vi "DrawBarPlot.vi"(0 "reference in":refnum<class "LcWebView.lvclass">, 1 "XLabels":string[](array[string]), 2 "BarPlot.Dataset":dbl[][](array[numeric]), 3 "BarPlot.DatasetLabels":string[](array[string]), 5 "Error In":errorcluster, 6 "GenericPlotOptions":T2, 7 "BarPlot.PlotColours":u32[](array[numeric]), 8 "BarPlotOptions":T1={"xLabel"="", "yLabel"="", "DisplayXLabel"=TRUE, "DisplayYLabel"=TRUE, "Stacked"=TRUE}) -> (14 "reference out":refnum<class "LcWebView.lvclass">, 19 "Error Out":errorcluster)   [LabVIEW 2020, in "LcWebView.lvclass"]
uses:
  LcWebView.lvclass
  ctrls/GenericPlotOption.ctl
  <userlib>/_LabVIEWCommon/LcHTMLPlot/HTMLPlot_class/Controls/LegendPosition.ctl
  ctrls/BarPlotOption.ctl
  <userlib>/_LabVIEWCommon/LcHTMLPlot/HTMLPlot_class/Controls/GenericPlotOptions.ctl
  <userlib>/_LabVIEWCommon/LcHTMLPlot/HTMLPlot_class/Controls/BarPlotOptions.ctl
  cdfa7b6c-348e-4618-b79e-b8b55caa0d01.vi
  <vilib>/JDP Science/JSONtext/Variant to JSON Text.vi
  <vilib>/JDP Science/JSONtext/LVClass Serializer/JSONtext LVClass Serializer.lvclass
  <userlib>/_LabVIEWCommon/LcHTMLPlot/HTMLPlot_class/HTMLPlot.lvclass
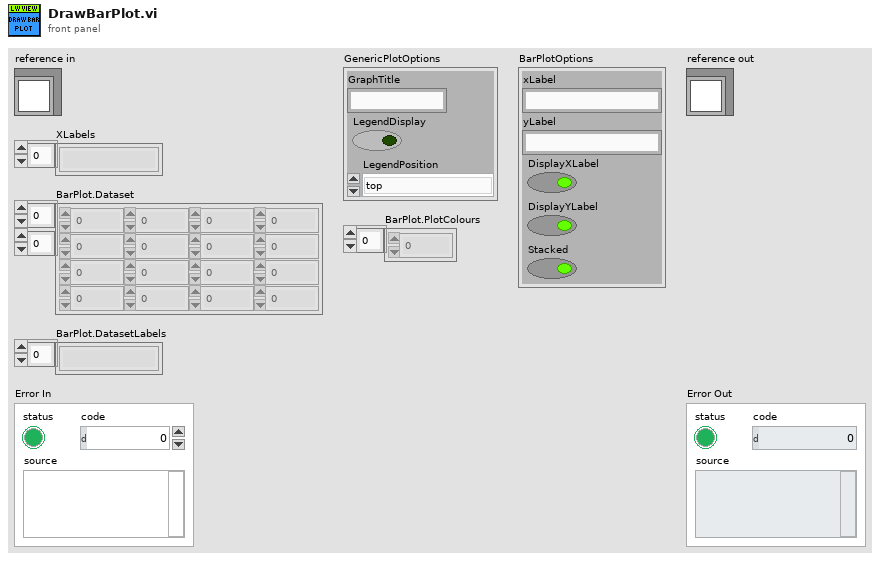
[diagram p1: front panel]
types:
  T1 = typedef "LcWebView.lvclass/BarPlotOption.ctl" = cluster{"xLabel":string, "yLabel":string, "DisplayXLabel":bool, "DisplayYLabel":bool, "Stacked":bool}
  T2 = typedef "LcWebView.lvclass/GenericPlotOption.ctl" = cluster{"GraphTitle":string, "LegendDisplay":bool, "LegendPosition":T3}
  T3 = typedef "HTMLPlot.lvclass/LegendPosition.ctl" = enum16{"top", "right", "left", "bottom"}
  T4 = typedef "HTMLPlot.lvclass/GenericPlotOptions.ctl" = cluster{"GraphTitle":string, "LegendDisplay":bool, "LegendPosition":T3}
  T5 = typedef "HTMLPlot.lvclass/BarPlotOptions.ctl" = cluster{"xLabel":string, "yLabel":string, "DisplayXLabel":bool, "DisplayYLabel":bool, "Stacked":bool}
  T6 = cluster{"action":string, "PlotData":string, "GenericPlotOptions":T4, "BarPlotOptions":T5}
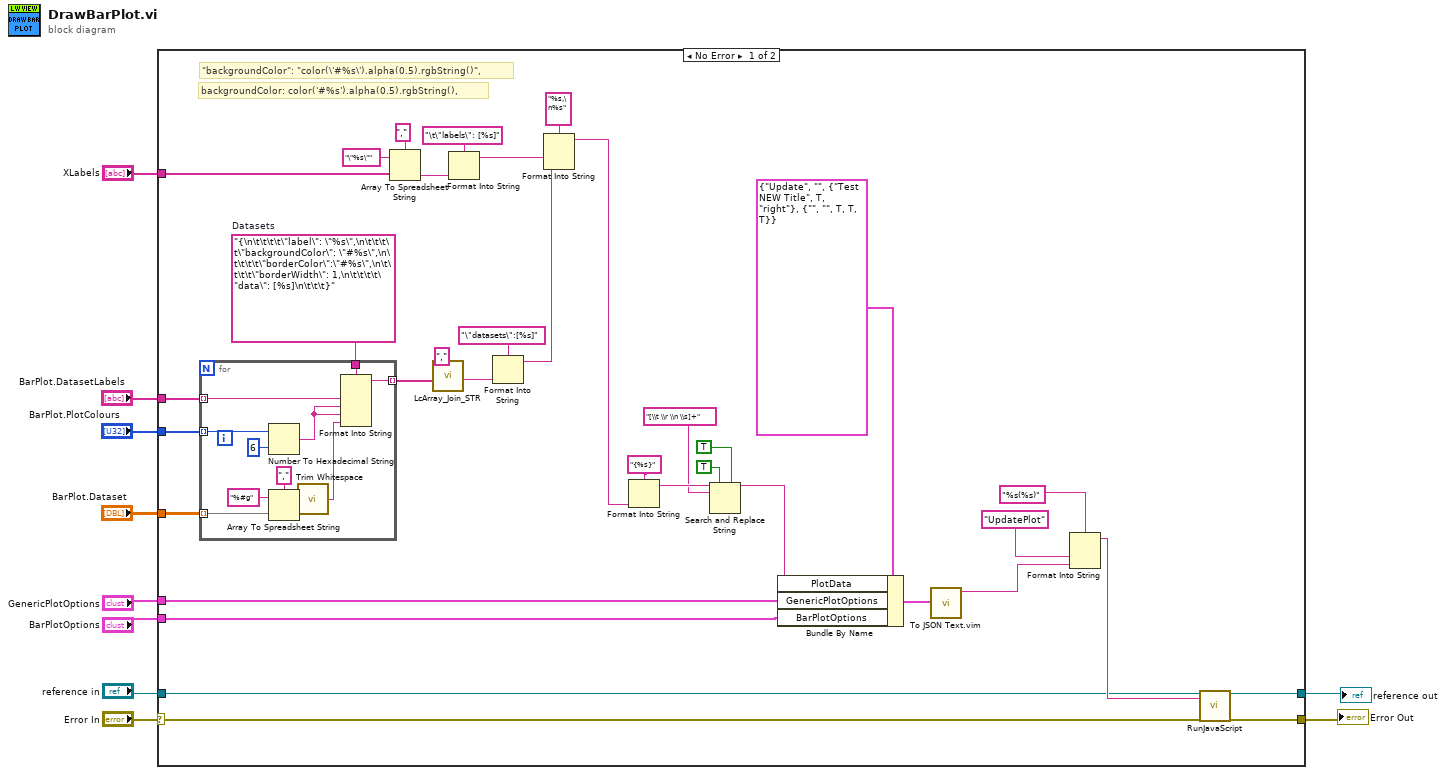
[diagram p0: block diagram]
diagram:
  n1 = case shown="No Error" "Error In" {
    selector: "Error In" -> [w11 w58]
    tunnel: [w12 w58] -> w1
    tunnel: [w13 w57] -> w2
    tunnel: "reference in" -> [w14 w57]
    tunnel: "BarPlot.Dataset" -> [w33 _]
    tunnel: "BarPlot.PlotColours" -> [w32 _]
    tunnel: "BarPlot.DatasetLabels" -> [w31 _]
    tunnel: "XLabels" -> [w30 _]
    tunnel: "GenericPlotOptions" -> [w22 _]
    tunnel: "BarPlotOptions" -> [w21 _]
    frame No Error {
      w34 = "{\n\t\t\t\t\"label\": \"%s\",\n\t\t\t\t\"backgroundColor\": \"#%s\",\n\t\t\t\t\"borderColor\":\"#%s\",\n\t\t\t\t\"borderWidth\": 1,\n\t\t\t\t\"data\": [%s]\n\t\t\t}"  # Datasets
      # "\"backgroundColor\": \"color(\\'#%s\\').alpha(0.5).rgbString()\","
      # "backgroundColor: color('#%s').alpha(0.5).rgbString(),"
      n2 = for {
        tunnel: w33 -> [w54] mode=indexing
        tunnel: w32 -> [w50] mode=indexing
        tunnel: w31 -> [w52] mode=indexing
        tunnel: [w51] -> w39 mode=indexing
        tunnel: w34 -> [w53]
        n3 = Number To Hexadecimal String(1:i16 6 ("width (-)"), 2:w50) -> (0:w49:string)
        n4 = Array To Spreadsheet String(delimiter (Tab)=",", array=w54, 3:"%#g" ("format string")) -> (spreadsheet string=w48:string)
        n5 = call <vilib>:"Trim Whitespace.vi"("string"=w48) -> ("trimmed string"=w47:string)  [unwired: 1 in]
        n6 = Format Into String(format string=w53, w52, w49, w49, w47) -> (resulting string=w51:string)  [unwired: 2 in, 1 out]
      }
      n7 = Array To Spreadsheet String(delimiter (Tab)=",", array=w30, 3:"\"%s\"" ("format string")) -> (spreadsheet string=w41:string)
      n8 = call <userlib>:"LcArray_Join_STR.vi"("separator"=",", "Array"=w39) -> ("joined string"=w38:string)  [unwired: 8 in, 1 out]
      n9 = Format Into String(format string="\t\"labels\": [%s]", w41) -> (resulting string=w44:string)  [unwired: 2 in, 1 out]
      n10 = Format Into String(format string="\"datasets\":[%s]", w38) -> (resulting string=w36:string)  [unwired: 2 in, 1 out]
      n11 = Format Into String(format string="%s,\n%s", w44, w36) -> (resulting string=w28:string)  [unwired: 2 in, 1 out]
      n12 = Format Into String(format string="{%s}", w28) -> (resulting string=w27:string)  [unwired: 2 in, 1 out]
      n13 = Search and Replace String(replace all?=TRUE ("replace all? (F)"), multiline?=TRUE ("multiline? (F)"), input string=w27, search string="[\\t \\r \\n \\s]+") -> (result string=w26:string)  [unwired: 4 in, 3 out]
      n14 = Bundle By Name(cluster=T6 {"action"="Update", "PlotData"="", "GenericPlotOptions"={"GraphTitle"="Test NEW Title", "LegendDisplay"=TRUE, "LegendPosition"=enum."right"}, "BarPlotOptions"={"xLabel"="", "yLabel"="", "DisplayXLabel"=TRUE, "DisplayYLabel"=TRUE, "Stacked"=TRUE}}, "PlotData"=w26, "GenericPlotOptions"=w22, "BarPlotOptions"=w21) -> (w19:T6)
      n15 = call "To JSON Text.vim"("Anything"=w19) -> ("<JSON>"=w16:string)  [unwired: 9 in, 1 out]
      n16 = Format Into String(format string="%s(%s)", "UpdatePlot" ("input 1"), w16) -> (resulting string=w15:string)  [unwired: 2 in, 1 out]
      n17 = call-dynamic "RunJavaScript.vi"("reference in"=w14, "Java Script Function"=w15, "Error In"=w11) -> ("reference out"=w13:refnum<class "LcWebView.lvclass">, "Error Out"=w12:errorcluster)  [unwired: 13 in, 2 out]
    }
    frame Error {
    }
  }
  "Error Out" <- w1
  "reference out" <- w2
